vi "ma_sml_Window Frequency Response (double).vi"(1 "N (window length)":i32=512, 2 "window":u16(ring) items=["Rectangle"=0, "Hanning"=1, "Hamming"=2, "Blackman-Harris"=3, "Exact Blackman"=4, "Blackman"=5, "Flat Top"=6, "4 Term B-Harris "=7, "7 Term B-Harris"=8, "Low Sidelobe"=9, "Blackman Nuttall"=11, "Triangle"=30, "Bartlett-Hanning"=31, "Bohman"=32, "Parzen"=33, "Welch"=34, "Kaiser"=60, "Dolph-Chebyshev"=61, "Gaussian"=62], 3 "f(normalized)":dbl format="%.5f") -> (0 "H(f)":cdb format="%.5e")   [LabVIEW 2020, in "NI_MAPro.lvlib"]
uses:
  NI_MAPro.lvlib
  <resource>/lvanlys.dll
panel:
  out "window properties":cluster{"eq noise BW":dbl, "coherent gain":dbl}
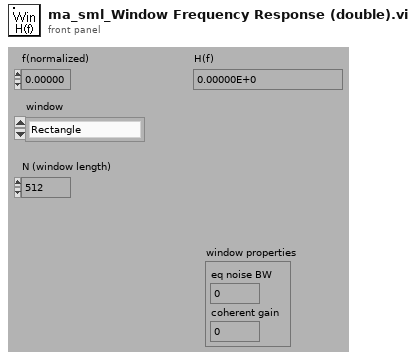
[diagram p1: front panel]
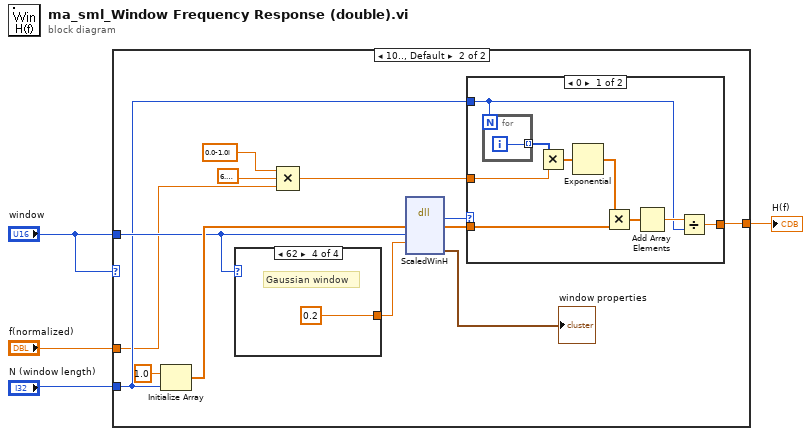
[diagram p0: block diagram]
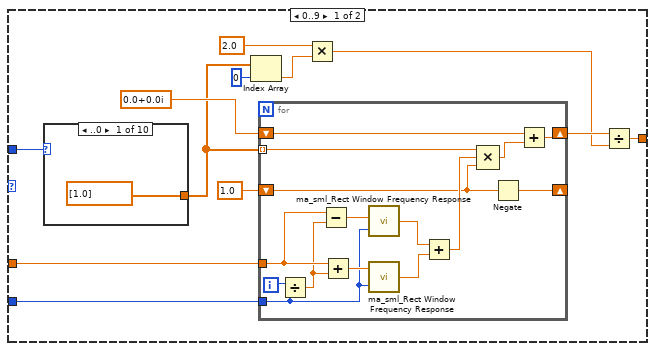
[diagram p2: hidden frame]
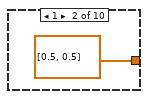
[diagram p3: hidden frame]
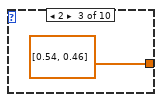
[diagram p4: hidden frame]
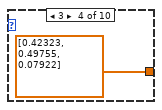
[diagram p5: hidden frame]
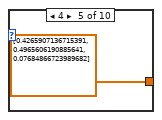
[diagram p6: hidden frame]
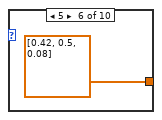
[diagram p7: hidden frame]
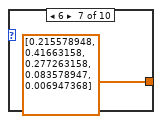
[diagram p8: hidden frame]
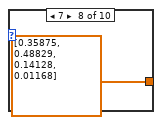
[diagram p9: hidden frame]
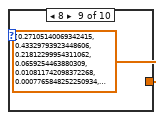
[diagram p10: hidden frame]
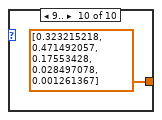
[diagram p11: hidden frame]
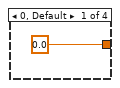
[diagram p13: hidden frame]
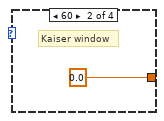
[diagram p14: hidden frame]
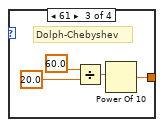
[diagram p15: hidden frame]
diagram:
  n1 = case shown="10.., Default" "window" {
    tunnel: "f(normalized)" -> [w10 w45]
    tunnel: "window" -> [w6 w51]
    tunnel: "N (window length)" -> [w9 w47]
    tunnel: [w7 w46] -> w2
    frame 0..9 {
      n2 = case shown="..0" w6 {
        tunnel: [dbl[] [1.0] ("Array") dbl[] [0.5, 0.5] ("Array") dbl[] [0.54, 0.46] ("Array") dbl[] [0.42323, 0.49755, 0.07922] ("Array") dbl[] [0.4265907136715391, 0.4965606190885641, 0.07684866723989682] ("Array") dbl[] [0.42, 0.5, 0.08] ("Array") dbl[] [0.215578948, 0.41663158, 0.277263158, 0.083578947, 0.006947368] ("Array") dbl[] [0.35875, 0.48829, 0.14128, 0.01168] ("Array") dbl[] [0.27105140069342415, 0.43329793923448606, 0.21812299954311062, 0.0659254463880309, 0.010811742098372268, 0.0007765848252250934, 1.3887217350903198e-05] ("Array") dbl[] [0.323215218, 0.471492057, 0.17553428, 0.028497078, 0.001261367] ("Output Array")] -> w5
        frame ..0 {
        }
        frame 1 {
        }
        frame 2 {
        }
        frame 3 {
        }
        frame 4 {
        }
        frame 5 {
        }
        frame 6 {
        }
        frame 7 {
        }
        frame 8 {
        }
        frame 9.. {
        }
      }
      n3 = Index Array(array=w5, index=0 ("Index")) -> (element=w12:dbl)
      n4 = for {
        tunnel: w5 -> [w38] mode=indexing
        tunnel: w10 -> [w35]
        tunnel: w9 -> [w31]
        shift-right: [w39] -> w15
        shift-left: cdb 0.0+0.0i -> [w40]
        shift-right: [w28] -> _
        shift-left: 1.0 ("y") -> [w27]
        i -> [w41]
        n5 = Divide(x=w41, y=w31) -> (x/y=w34:dbl)
        n6 = Subtract(x=w35, y=w34) -> (x-y=w32:dbl)
        n7 = Add(x=w35, y=w34) -> (x+y=w33:dbl)
        n8 = call "ma_sml_Rect Window Frequency Response.vi"("N"=w31, "f"=w32) -> ("H(f)"=w30:cdb)
        n9 = call "ma_sml_Rect Window Frequency Response.vi"("N"=w31, "f"=w33) -> ("H(f)"=w29:cdb)
        n10 = Add(x=w30, y=w29) -> (x+y=w37:cdb)
        n11 = Compound Arithmetic op=MULTIPLY(w38, w37, w27) -> (w36:cdb)
        n12 = Negate(x=w27) -> (-x=w28:dbl)
        n13 = Add(x=w40, y=w36) -> (x+y=w39:cdb)
      }
      n14 = Multiply(x=2.0 ("y"), y=w12) -> (x*y=w11:dbl)
      n15 = Divide(x=w15, y=w11) -> (x/y=w7:cdb)
    }
    frame 10.., Default {
      n16 = Initialize Array(1.0 ("element"), w47) -> (w52:dbl[])
      n17 = case shown="62" w51 {
        tunnel: [0.0 ("s(db)") 0.0 w68 0.2 ("para")] -> w53
        frame 0, Default {
        }
        frame 60 {
          # "Kaiser window"
        }
        frame 61 {
          # "Dolph-Chebyshev"
          n18 = Divide(x=60.0 ("y"), y=20.0) -> (x/y=w69:dbl)
          n19 = Power Of 10(x=w69) -> (10^x=w68:dbl)
        }
        frame 62 {
          # "Gaussian window"
        }
      }
      n20 = Compound Arithmetic op=MULTIPLY(cdb 0.0-1.0i, 6.283185307179586, w45) -> (w44:cdb)
      n21 = dll-call lib="C:/Program Files (x86)/National Instruments/LabVIEW 2020/resource/lvanlys.*" fn="ScaledWinH"("xH"=w52, "winType"=w51, "para"=w53) -> ("return type"=w49:i32, "xH"=w48:dbl[], "window properties"=→"window properties":cluster{"eq noise BW":dbl, "coherent gain":dbl})  [unwired: 5 in, 3 out]
      n22 = case shown="0" w49 {
        tunnel: w48 -> [w62 _]
        tunnel: w47 -> [w59 _]
        tunnel: w44 -> [w56 _]
        tunnel: [w58 _] -> w46
        frame 0 {
          n23 = for {
            N: w59 -> [_]
            tunnel: [w64] -> w57 mode=indexing
            i -> [w64]
          }
          n24 = Multiply(x=w57, y=w56) -> (x*y=w55:cdb[])
          n25 = Exponential(1:w55) -> (0:w63:cdb[])
          n26 = Multiply(x=w63, y=w62) -> (x*y=w61:cdb[])
          n27 = Add Array Elements(numeric array=w61) -> (sum=w60:cdb)
          n28 = Divide(x=w60, y=w59) -> (x/y=w58:cdb)
        }
        frame 1, Default {
        }
      }
    }
  }
  "H(f)" <- w2
